vi "Part 1.vi"(11 "Input":string) -> (3 "Output":i64)   [LabVIEW 2021]
uses:
  <userlib>/_OpenG.lib/string/string.llb/Convert EOLs (String)__ogtk.vi
panel:
  out "array":string[](array[string])
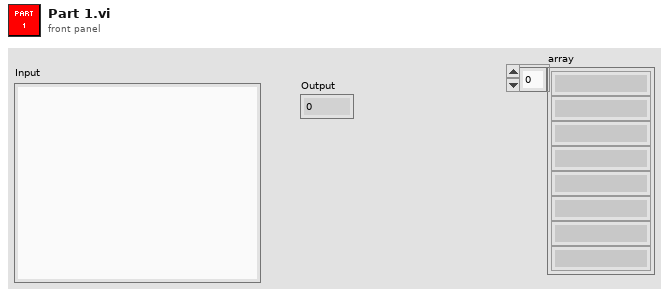
[diagram p1: front panel]
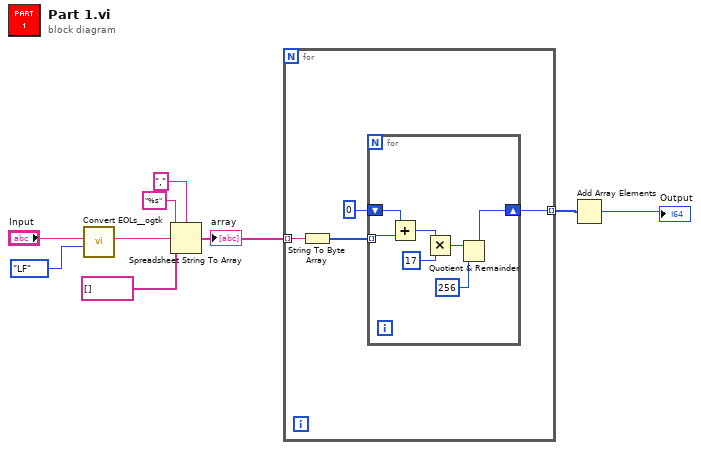
[diagram p0: block diagram]
diagram:
  n1 = call-poly <userlib>:"Convert EOLs__ogtk.vi"("Convert to:"=enum16{"CR", "LF", "CRLF"}."LF", "String in"="Input") -> ("String out"=w5:string)  [unwired: 9 in]
  n2 = Spreadsheet String To Array(delimiter (Tab)=",", format string="%s", spreadsheet string=w5, array type (2D Dbl)=string[] []) -> (array=w3:string[])
  "array" <- w3
  n3 = for {
    tunnel: w3 -> [w13] mode=indexing
    tunnel: [w10] -> w2 mode=indexing
    n4 = String To Byte Array(string=w13) -> (unsigned byte array=w12:u8[])
    n5 = for {
      tunnel: w12 -> [w20] mode=indexing
      shift-right: [w14] -> w10
      shift-left: 0 -> [w19]
      n6 = Add(x=w19, y=w20) -> (x+y=w18:i32)
      n7 = Multiply(x=w18, y=17) -> (x*y=w16:i32)
      n8 = Quotient & Remainder(x=w16, y=256) -> (x-y*floor(x/y)=w14:i32)  [unwired: 1 out]
    }
  }
  n9 = Add Array Elements(numeric array=w2) -> (sum=→"Output":i32)
